vi "Test Control Panel.vi"() -> ()   [LabVIEW 2017]
panel:
  out "Ready":bool
  out "PEM Name":string
  in  "wavelength":dbl[unit] min=0.0 max=1.99999e-05 step=1.0000000000000002e-10
  in  "Retardation 2":dbl=1.0 min=0.0 max=1.0 step=0.001
  in  "Set Retardation":bool
  in  "Set Wavelength":bool
  out "query output":string
  in  "Inhibit":bool
  out "Retardation":dbl
  out "Wavelength":dbl[unit]
  out "Frequency output":string
  out "Inhibited output":string
  in  "stop":bool
  out "VISA resource name out":refnum<visa-resource-name>
  out "error out":errorcluster
  in  "VISA resource name":refnum<visa-resource-name>="COM3"
  in  "error in (no error)":errorcluster
  # "On"
  # "Off"
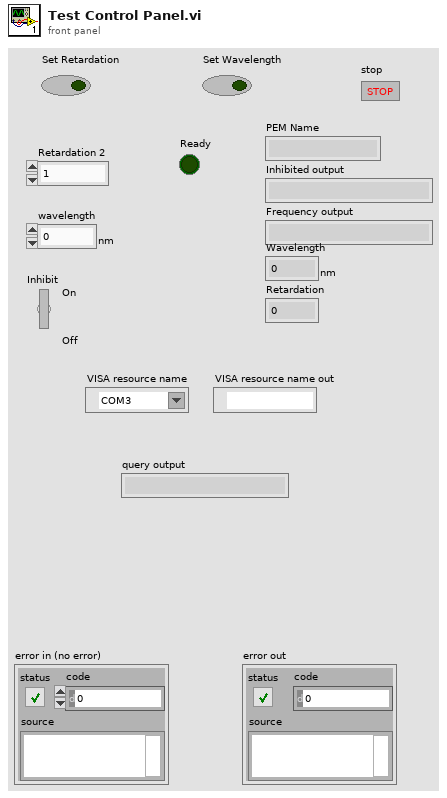
[diagram p1: front panel]
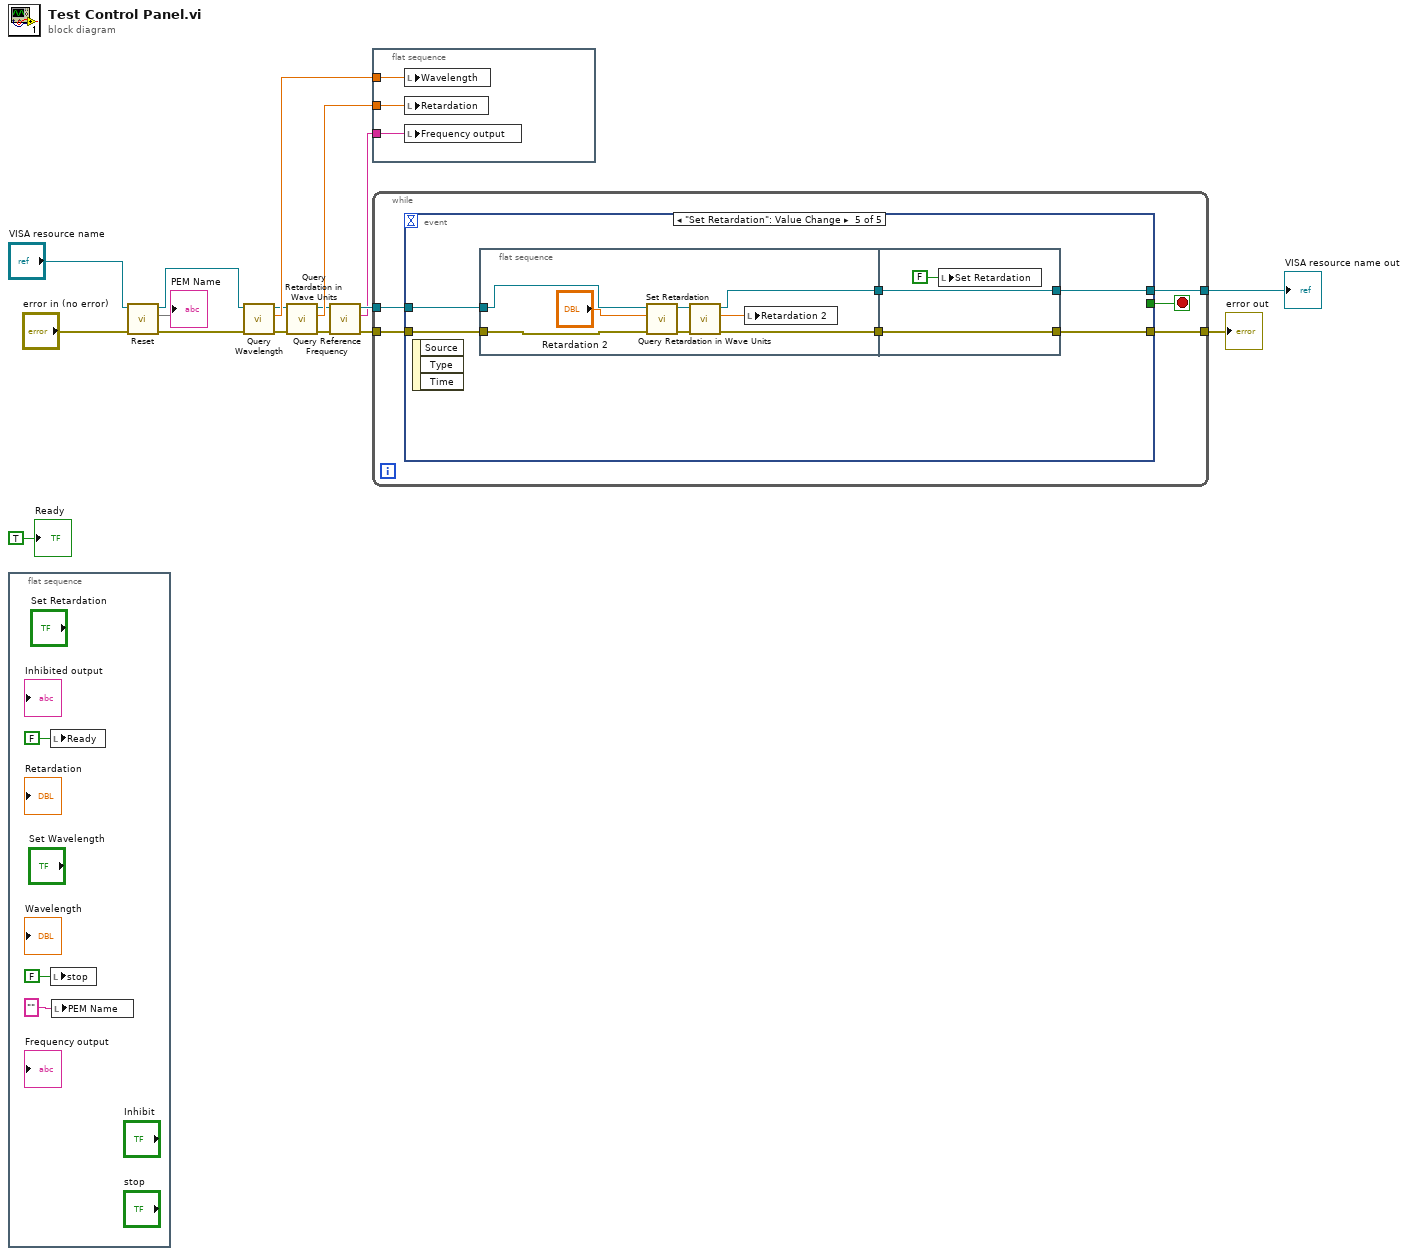
[diagram p0: block diagram]
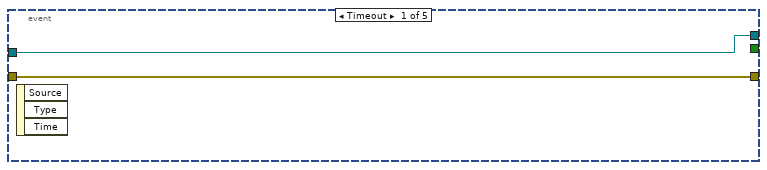
[diagram p2: hidden frame]
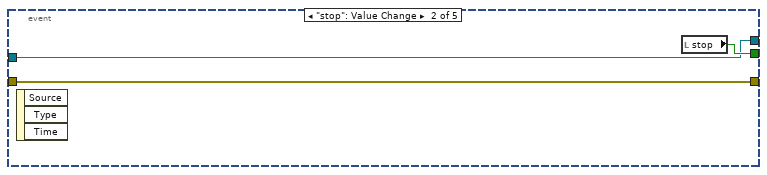
[diagram p3: hidden frame]
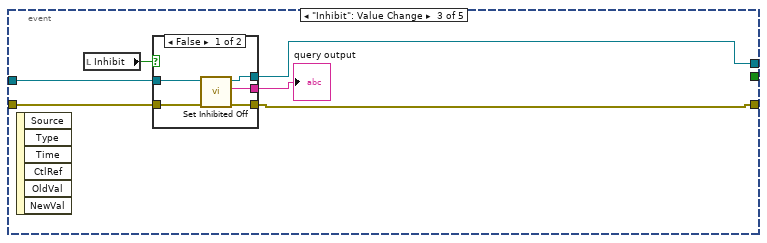
[diagram p4: hidden frame]
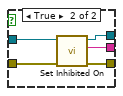
[diagram p5: hidden frame]
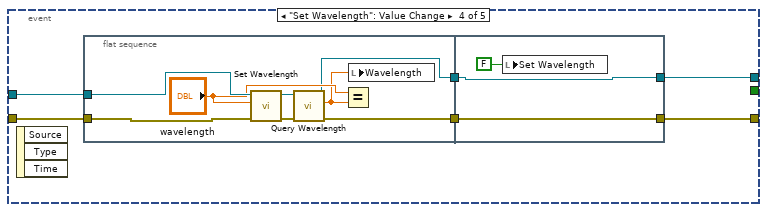
[diagram p6: hidden frame]
diagram:
  n1 = flat-sequence {
    frame #0 {
      n2 = local write "Ready"(FALSE ("Ready")) -> ()
      n3 = local write "stop"(FALSE ("stop")) -> ()
      n4 = local write "PEM Name"("" ("PEM Name")) -> ()
    }
  }
  n5 = call "Reset.vi"("error in (no error)"="error in (no error)", "VISA resource name"="VISA resource name") -> ("error out"=w8:errorcluster, 2:→"PEM Name", "VISA resource name out"=w7:refnum<visa-resource-name>)  [unwired: 7 in]
  n6 = call "Query Wavelength.vi"("error in (no error)"=w8, "VISA resource name"=w7) -> ("error out"=w5:errorcluster, "Wavelength"=w10:dbl[unit], "VISA resource name out"=w4:refnum<visa-resource-name>)  [unwired: 7 in]
  n7 = call "Query Retardation in Wave Units.vi"("error in (no error)"=w5, "VISA resource name"=w4) -> ("error out"=w2:errorcluster, "Fraction of wave Retardation"=w12:dbl, "VISA resource name out"=w3:refnum<visa-resource-name>)  [unwired: 7 in]
  n8 = call "Query Reference Frequency.vi"("error in (no error)"=w2, "VISA resource name"=w3) -> ("error out"=w13:errorcluster, "Frequency output"=w9:string, "VISA resource name out"=w11:refnum<visa-resource-name>)  [unwired: 7 in]
  n9 = flat-sequence {
    tunnel: w12 -> [w23]
    tunnel: w10 -> [w21]
    tunnel: w9 -> [w22]
    frame #0 {
      n10 = local write "Wavelength"(w21) -> ()
      n11 = local write "Retardation"(w23) -> ()
      n12 = local write "Frequency output"(w22) -> ()
    }
  }
  n13 = while {
    tunnel: [w28] -> w15
    tunnel: [w27] -> w14
    tunnel: w13 -> [w25]
    tunnel: w11 -> [w24]
    stop <- w26 stop-if-true
    n14 = event shown="[4] \"Set Retardation\": Value Change" {
      selector: _ -> [_ _ _ _ _]
      dyn-events: _ -> [_ _ _ _ _]
      timeout: _ -> [_ _ _ _ _]
      tunnel: w25 -> [w30 w32 w34 w54 w72]
      tunnel: w24 -> [w29 w31 w35 w55 w71]
      tunnel: [w30 w32 w38 w52 w69] -> w28
      tunnel: [w29 w31 w39 w53 w70] -> w27
      tunnel: [_ w33 _ _ _] -> w26
      event Timeout {
        n15 = event-data() -> ()  [unwired: 1 in, 3 out]
      }
      event "stop": Value Change {
        n16 = event-data() -> ()  [unwired: 1 in, 3 out]
        n17 = local read "stop"() -> (w33:bool)
      }
      event "Inhibit": Value Change {
        n18 = event-data() -> ()  [unwired: 1 in, 6 out]
        n19 = local read "Inhibit"() -> (w37:bool)
        n20 = case shown="False" w37 {
          tunnel: w34 -> [w43 w49]
          tunnel: w35 -> [w44 w48]
          tunnel: [w42 w47] -> w38
          tunnel: [w40 w46] -> w36
          tunnel: [w41 w45] -> w39
          frame False {
            n21 = call "Set Inhibited Off.vi"("error in (no error)"=w43, "VISA resource name"=w44) -> ("error out"=w42:errorcluster, "query output"=w40:string, "VISA resource name out"=w41:refnum<visa-resource-name>)  [unwired: 7 in]
          }
          frame True {
            n22 = call "Set Inhibited On.vi"("error in (no error)"=w49, "VISA resource name"=w48) -> ("error out"=w47:errorcluster, "query output"=w46:string, "VISA resource name out"=w45:refnum<visa-resource-name>)  [unwired: 7 in]
          }
        }
        "query output" <- w36
      }
      event "Set Wavelength": Value Change {
        n23 = event-data() -> ()  [unwired: 1 in, 3 out]
        n24 = flat-sequence {
          tunnel: w55 -> [w63]
          tunnel: w54 -> [w62]
          tunnel: [w60] -> w51
          tunnel: [w59] -> w50
          tunnel: [w65] -> w52
          tunnel: [w66] -> w53
          tunnel: w51 -> [w66]
          tunnel: w50 -> [w65]
          frame #0 {
            n25 = call "Set Wavelength.vi"("error in (no error)"=w62, "wavelength"="wavelength", "VISA resource name"=w63) -> ("error out"=w56:errorcluster, "VISA resource name out"=w57:refnum<visa-resource-name>)  [unwired: 5 in, 2 out]
            n26 = call "Query Wavelength.vi"("error in (no error)"=w56, "VISA resource name"=w57) -> ("error out"=w59:errorcluster, "Wavelength"=w58:dbl[unit], "VISA resource name out"=w60:refnum<visa-resource-name>)  [unwired: 7 in]
            n27 = Equal?(x="wavelength", y=w58) -> ()  [unwired: 1 out]
            n28 = local write "Wavelength"(w58) -> ()
          }
          frame #1 {
            n29 = local write "Set Wavelength"(FALSE ("Set Wavelength")) -> ()
          }
        }
      }
      event "Set Retardation": Value Change {
        n30 = event-data() -> ()  [unwired: 1 in, 3 out]
        n31 = flat-sequence {
          tunnel: w72 -> [w79]
          tunnel: w71 -> [w78]
          tunnel: [w75] -> w68
          tunnel: [w73] -> w67
          tunnel: [w82] -> w69
          tunnel: [w83] -> w70
          tunnel: w68 -> [w83]
          tunnel: w67 -> [w82]
          frame #0 {
            n32 = call "Set Retardation.vi"("error in (no error)"=w79, "Retardation"="Retardation 2", "VISA resource name"=w78) -> ("error out"=w74:errorcluster, "VISA resource name out"=w76:refnum<visa-resource-name>)  [unwired: 6 in, 1 out]
            n33 = call "Query Retardation in Wave Units.vi"("error in (no error)"=w74, "VISA resource name"=w76) -> ("error out"=w73:errorcluster, "Fraction of wave Retardation"=w77:dbl, "VISA resource name out"=w75:refnum<visa-resource-name>)  [unwired: 7 in]
            n34 = local write "Retardation 2"(w77) -> ()
          }
          frame #1 {
            n35 = local write "Set Retardation"(FALSE ("Set Retardation")) -> ()
          }
        }
      }
    }
  }
  "error out" <- w15
  "VISA resource name out" <- w14
  "Ready" <- TRUE ("Ready")
